vi "uActor_Core.vi"(8 "error in (no error)":errorcluster, 11 "uActor in":refnum<class "uActor.lvclass">) -> (0 "error out":errorcluster, 3 "uActor out":refnum<class "uActor.lvclass">)   [LabVIEW 2023, in "uFramework.lvlib" / "uActor.lvclass"]
doc: "Dynamic dispatch method to allow children to add helper loops when desired."
uses:
  uActor.lvclass
  uActor.lvclass/uActor.ctl
  uTransport_uActor/uTransport_uActor.lvclass
  uMsg/uMsg.lvclass
  Bin/uData.lvlibp/uData.lvclass
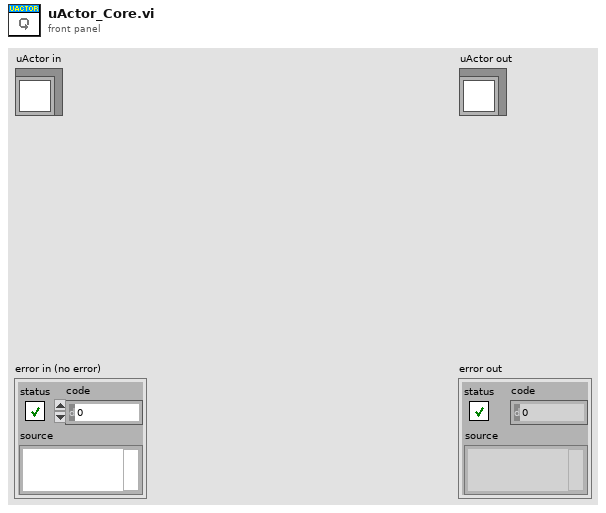
[diagram p1: front panel]
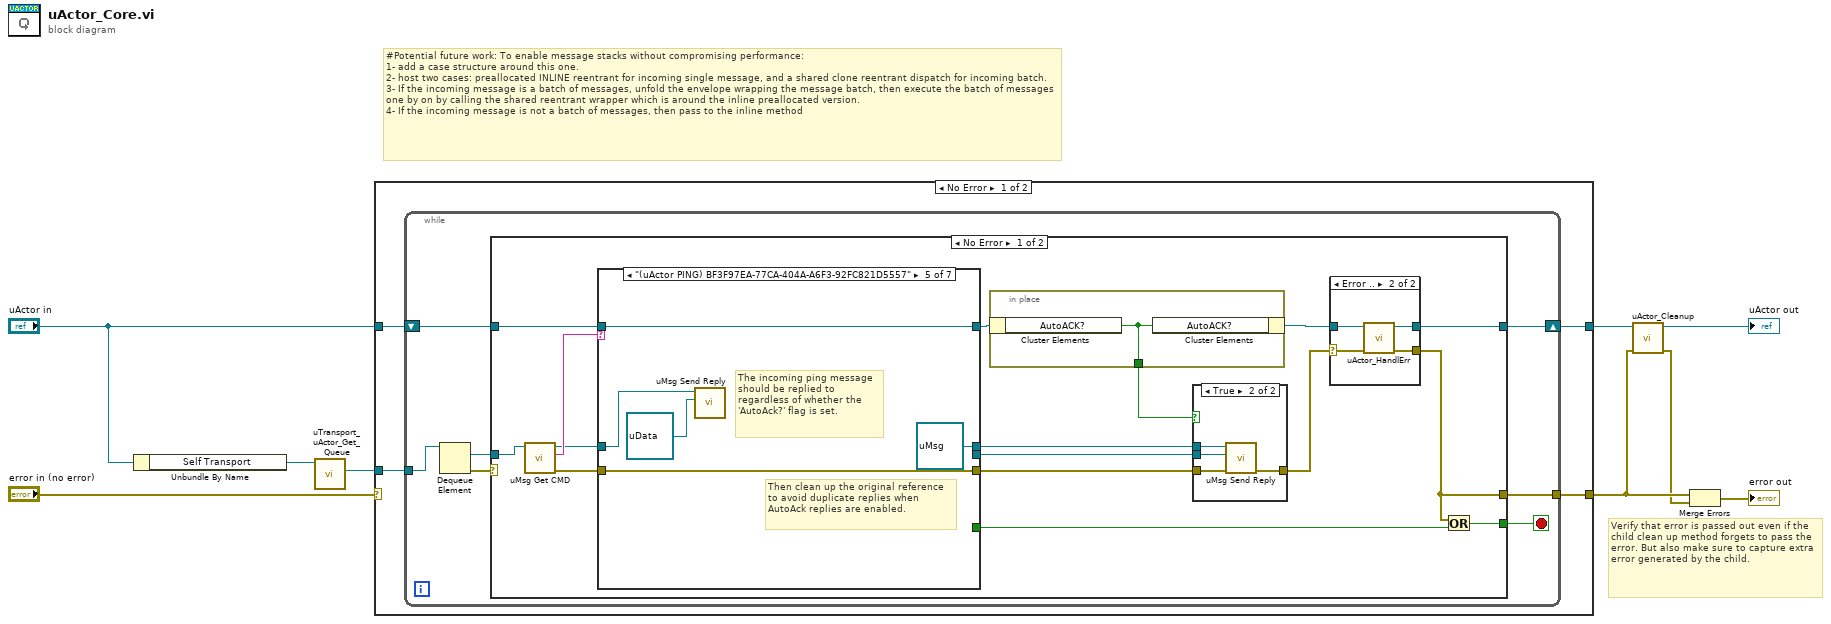
[diagram p0: block diagram]
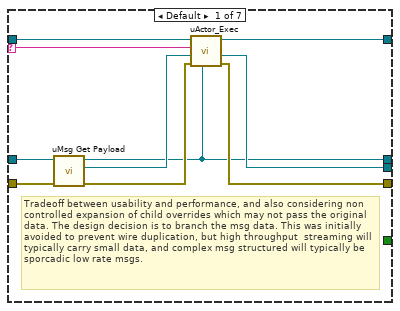
[diagram p2: hidden frame]
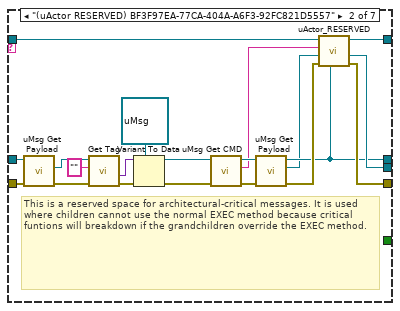
[diagram p3: hidden frame]
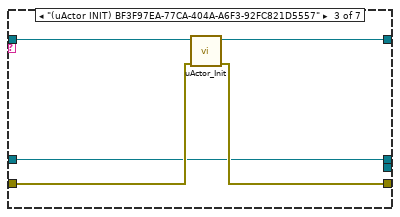
[diagram p4: hidden frame]
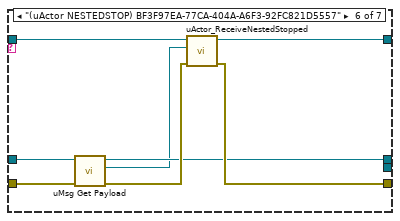
[diagram p6: hidden frame]
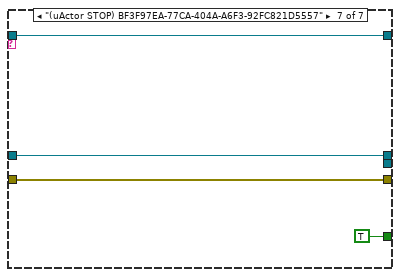
[diagram p7: hidden frame]
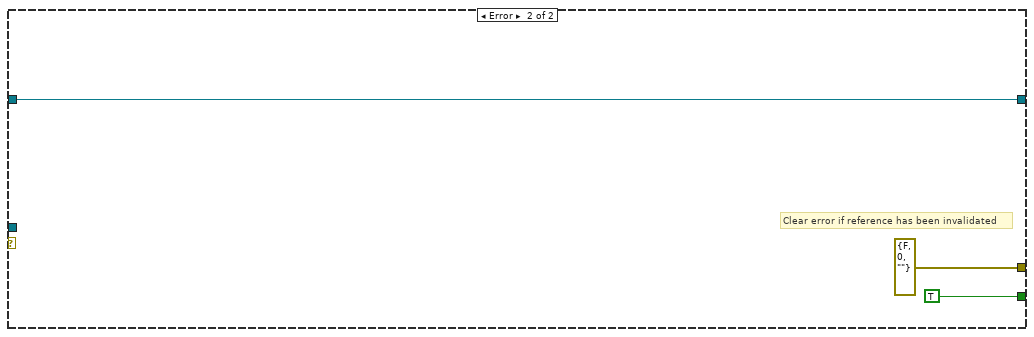
[diagram p10: hidden frame]
diagram:
  # "Verify that error is passed out even if the child clean up method forgets to pass the error. But also make sure to capture extra error generated by the child."
  # "#Potential future work: To enable message stacks without compromising performance:\n1- add a case structure around this one. \n2- host two cases: preallocated INLINE reentrant for incoming single message, and a shared clone reentrant dispatch for incoming batch.\n3- If the incoming message is a batch of messages, unfold the envelope wrapping the message batch, then execute the batch of messages one by on by calling the shared reentrant wrapper which is around the inline preallocated version.\n4- If the incoming message is not a batch of messages, then pass to the inline method"
  n1 = Unbundle By Name("uActor in") -> ("Self Transport"=w8:refnum<class "uTransport_uActor.lvclass">)
  n2 = call "uTransport_uActor_Get_Queue.vi"("uTransport_uActor in"=w8) -> ("Actor Queue"=w7:refnum<queue>)  [unwired: 10 in]
  n3 = case shown="No Error" "error in (no error)" {
    selector: "error in (no error)" -> [_ w108]
    tunnel: [w10 w108] -> w3
    tunnel: [w13 w107] -> w6
    tunnel: "uActor in" -> [w12 w107]
    tunnel: w7 -> [w11 _]
    frame No Error {
      n4 = while {
        shift-right: [w17] -> w13
        shift-left: w12 -> [w19]
        tunnel: w11 -> [w20]
        tunnel: [w15] -> w10
        stop <- w16 stop-if-true
        n5 = Dequeue Element(queue=w20) -> (element=w18:refnum<class "uMsg.lvclass">, error out=w14:errorcluster)  [unwired: 2 in, 2 out]
        n6 = case shown="No Error" w14 {
          tunnel: w19 -> [w35 w104]
          tunnel: w18 -> [w34 _]
          tunnel: [w32 w104] -> w17
          tunnel: [w31 TRUE] -> w16
          tunnel: [w30 errorcluster {"status"=FALSE, "code"=0, "source"=""} ("error out")] -> w15
          frame No Error {
            n7 = call "uMsg Get CMD.vi"("uMsg in"=w34) -> ("error out"=w36:errorcluster, "CMD"=w33:string, "uMsg out"=w26:refnum<class "uMsg.lvclass">)  [unwired: 8 in]
            n8 = case shown="\"(uActor PING) BF3F97EA-77CA-404A-A6F3-92FC821D5557\"" w33 {
              selector: w33 -> [w44 _ _ _ _ _ _]
              tunnel: [w45 w65 w70 w74 w79 w86 w90] -> w28
              tunnel: w36 -> [w41 w63 w69 w74 w79 w83 w90]
              tunnel: [w47 w67 w72 w75 w80 w87 w91] -> w23
              tunnel: w35 -> [w46 w66 w71 w75 w80 w88 w91]
              tunnel: w26 -> [w40 w62 w68 w73 w78 w85 w89]
              tunnel: [_ _ _ _ _ _ TRUE] -> w29
              tunnel: [w43 w64 _ _ _ _ _] -> w27
              tunnel: [w38 w53 w68 w73 refnum<class "uMsg.lvclass"> refnum ("uMsg out") w82 w89] -> w25
              frame Default {
                # "Tradeoff between usability and performance, and also considering non controlled expansion of child overrides which may not pass the original data. The design decision is to branch the msg data. This was initially avoided to prevent wire duplication, but high throughput  streaming will typically carry small data, and complex msg structured will typically be sporcadic low rate msgs."
                n9 = call "uMsg Get Payload.vi"("error in (no error)"=w41, "uMsg in"=w40) -> ("error out"=w42:errorcluster, "uData"=w39:refnum<class "uData.lvclass">, "uMsg out"=w38:refnum<class "uMsg.lvclass">)  [unwired: 7 in]
                n10 = call-dynamic "uActor_Exec.vi"("Original uMsg"=w38, "error in (no error)"=w42, "Data"=w39, "Command"=w44, "uActor in"=w46) -> ("error out"=w45:errorcluster, "reply"=w43:refnum<class "uData.lvclass">, "uActor out"=w47:refnum<class "uActor.lvclass">)  [unwired: 4 in]
              }
              frame "(uActor RESERVED) BF3F97EA-77CA-404A-A6F3-92FC821D5557" {
                # "This is a reserved space for architectural-critical messages. It is used where children cannot use the normal EXEC method because critical funtions will breakdown if the grandchildren override the EXEC method."
                n11 = call "uMsg Get Payload.vi"("error in (no error)"=w63, "uMsg in"=w62) -> ("error out"=w61:errorcluster, "uData"=w59:refnum<class "uData.lvclass">)  [unwired: 7 in, 1 out]
                n12 = call "Get Tag.vi"("error in (no error)"=w61, "tag (case insensitive)"="", "uData in"=w59) -> ("error out"=w60:errorcluster, "value"=w57:variant)  [unwired: 5 in, 2 out]
                n13 = Variant To Data(error in=w60, type=refnum<class "uMsg.lvclass"> refnum ("uMsg out"), Variant=w57) -> (data=w50:refnum<class "uMsg.lvclass">, error out=w55:errorcluster)
                n14 = call "uMsg Get CMD.vi"("error in (no error)"=w55, "uMsg in"=w50) -> ("error out"=w51:errorcluster, "CMD"=w48:string, "uMsg out"=w49:refnum<class "uMsg.lvclass">)  [unwired: 7 in]
                n15 = call "uMsg Get Payload.vi"("error in (no error)"=w51, "uMsg in"=w49) -> ("error out"=w54:errorcluster, "uData"=w52:refnum<class "uData.lvclass">, "uMsg out"=w53:refnum<class "uMsg.lvclass">)  [unwired: 7 in]
                n16 = call-dynamic "uActor_RESERVED.vi"("Original uMsg"=w53, "error in (no error)"=w54, "Data"=w52, "Command"=w48, "uActor in"=w66) -> ("error out"=w65:errorcluster, "reply"=w64:refnum<class "uData.lvclass">, "uActor out"=w67:refnum<class "uActor.lvclass">)  [unwired: 4 in]
              }
              frame "(uActor INIT) BF3F97EA-77CA-404A-A6F3-92FC821D5557" {
                n17 = call-dynamic "uActor_Init.vi"("error in (no error)"=w69, "uActor in"=w71) -> ("error out"=w70:errorcluster, "uActor out"=w72:refnum<class "uActor.lvclass">)  [unwired: 8 in]
              }
              frame "(uActor NULL) BF3F97EA-77CA-404A-A6F3-92FC821D5557" {
                # "Children may NOT override the blank string behavior. It invokes the the NULL case. Blank strings are part of the reserved non-overridable framework functions"
                # "Blank string received, or intentional NULL msg."
              }
              frame "(uActor PING) BF3F97EA-77CA-404A-A6F3-92FC821D5557" {
                # "Then clean up the original reference to avoid duplicate replies when AutoAck replies are enabled."
                # "The incoming ping message should be replied to regardless of whether the 'AutoAck?' flag is set."
                n18 = call "uMsg Send Reply.vi"("Reply Data"=refnum<class "uData.lvclass"> refnum, "Original Msg"=w78) -> ()  [unwired: 9 in, 1 out]
              }
              frame "(uActor NESTEDSTOP) BF3F97EA-77CA-404A-A6F3-92FC821D5557" {
                n19 = call "uMsg Get Payload.vi"("error in (no error)"=w83, "uMsg in"=w85) -> ("error out"=w84:errorcluster, "uData"=w81:refnum<class "uData.lvclass">, "uMsg out"=w82:refnum<class "uMsg.lvclass">)  [unwired: 7 in]
                n20 = call "uActor_ReceiveNestedStopped.vi"("error in (no error)"=w84, "uData in"=w81, "uActor in"=w88) -> ("error out"=w86:errorcluster, "uActor out"=w87:refnum<class "uActor.lvclass">)  [unwired: 7 in]
              }
              frame "(uActor STOP) BF3F97EA-77CA-404A-A6F3-92FC821D5557" {
              }
            }
            n21 = in-place {
              in-place-border: [w37] -> w21
              n22 = in-place-cluster #1(w23) -> ("AutoACK?"=w37:bool)
              n23 = in-place-cluster #1("AutoACK?"=w37) -> (w22:refnum<class "uActor.lvclass">)
            }
            n24 = case shown="True" w21 {
              tunnel: w28 -> [w93 w97]
              tunnel: w27 -> [_ w96]
              tunnel: w25 -> [_ w94]
              tunnel: [w93 w95] -> w24
              frame False {
              }
              frame True {
                n25 = call "uMsg Send Reply.vi"("error in (no error)"=w97, "Reply Data"=w96, "Original Msg"=w94) -> ("error out"=w95:errorcluster)  [unwired: 8 in]
              }
            }
            n26 = case shown="Error .." w24 {
              selector: w24 -> [w98 w101]
              tunnel: w22 -> [w99 w103]
              tunnel: [w99 w102] -> w32
              tunnel: [w98 w100] -> w30
              frame No Error {
              }
              frame Error {
                n27 = call "uActor_HandlErr.vi"("error in (no error)"=w101, "uActor in"=w103) -> ("error out"=w100:errorcluster, "uActor out"=w102:refnum<class "uActor.lvclass">)  [unwired: 8 in]
              }
            }
            n28 = Or(x=w30, y=w29) -> (x .or. y?=w31:bool)
          }
          frame Error {
            # "Clear error if reference has been invalidated"
          }
        }
      }
    }
    frame Error {
    }
  }
  n29 = call-dynamic "uActor_Cleanup.vi"("error in (no error)"=w3, "uActor in"=w6) -> ("error out"=w2:errorcluster, "uActor out"=→"uActor out":refnum<class "uActor.lvclass">)  [unwired: 8 in]
  n30 = Merge Errors(w3, w2) -> (→"error out":errorcluster)
